vi "自动升级程序.vi"(8 "错误输入（无错误）":errorcluster) -> (0 "错误输出":errorcluster, 3 "确定":bool)   [LabVIEW 2016, in "数据传输系统-04.lvlib" / "自动更新.lvlib"]
uses:
  <vilib>/Utility/miscctls.llb/LVPointTypeDef.ctl
panel:
  out "自动下载倒计时/s":i32
  in  "滚动条":i32(c297)
  out "标题":string
  in  "取消":bool
  in  "确定":bool
  out "版本说明显示":string
  # "是否立即下载新版本(download right now)?"
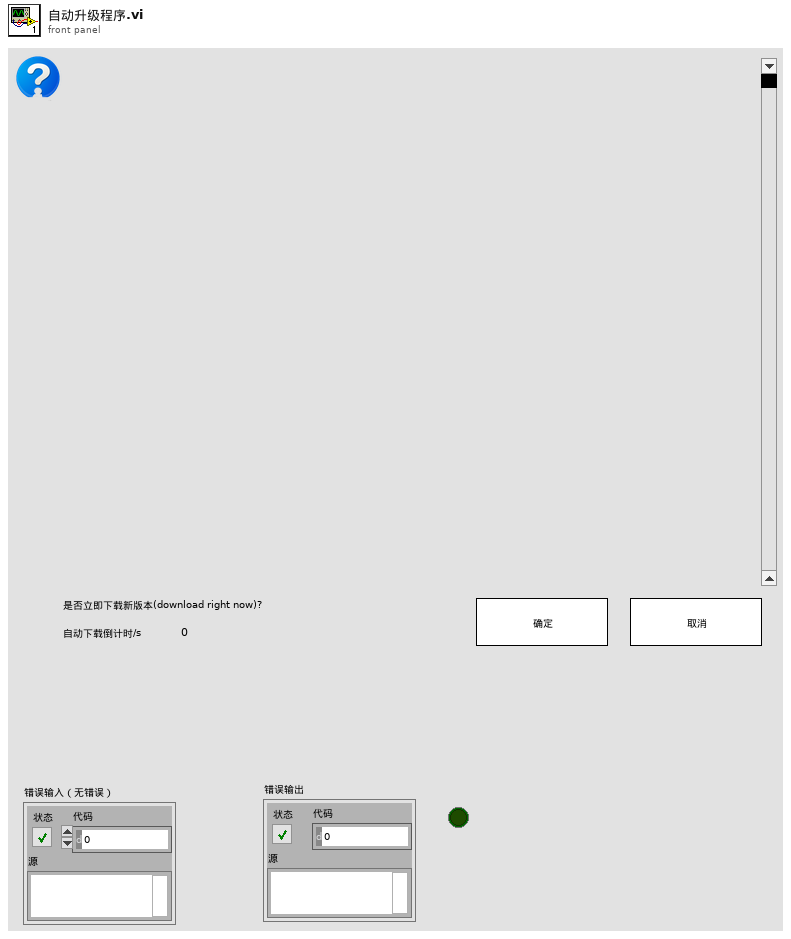
[diagram p1: front panel]
types:
  T1 = typedef "LVPointTypeDef.ctl" = cluster{"Horizontal":i16, "Vertical":i16}
  T2 = enum16{"open", "replace", "create", "open or create", "replace or create", "replace or create with confirmation"}
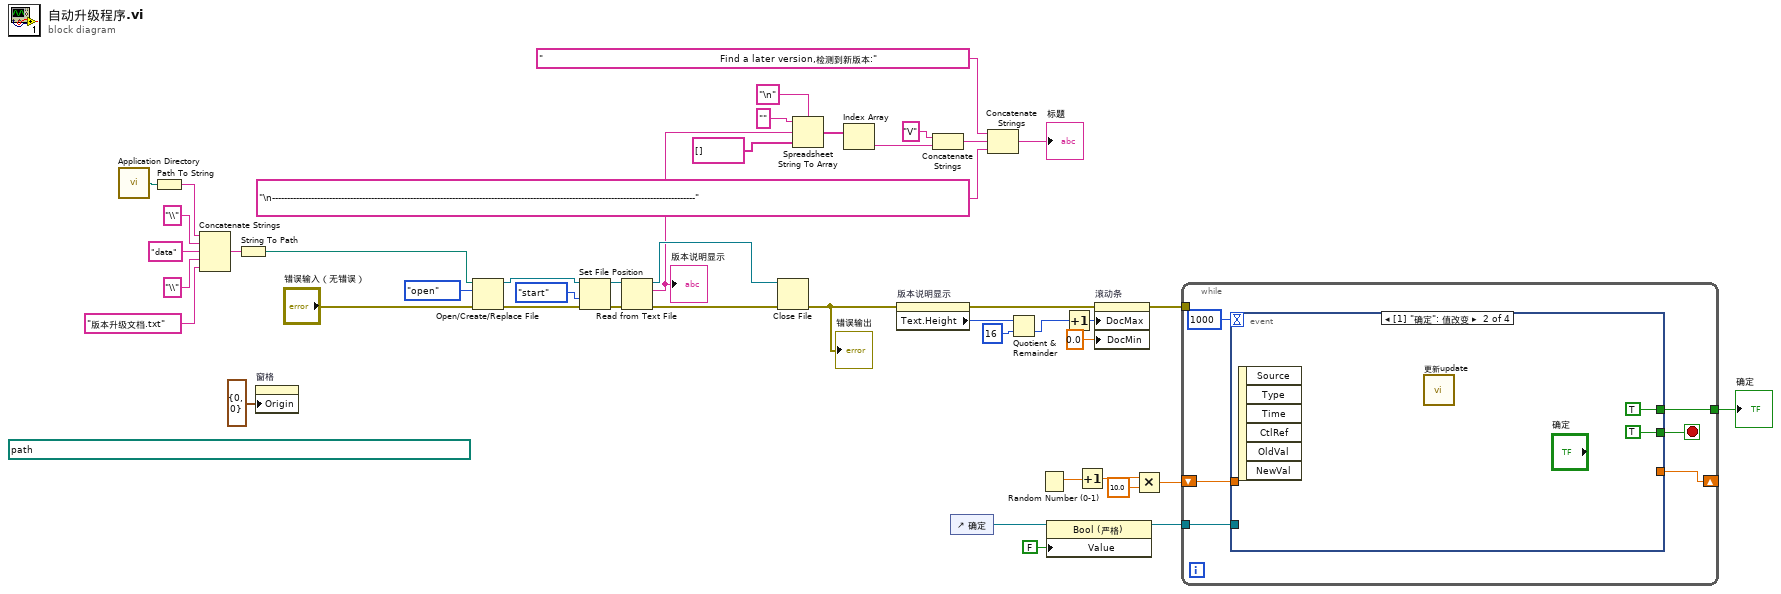
[diagram p0: block diagram]
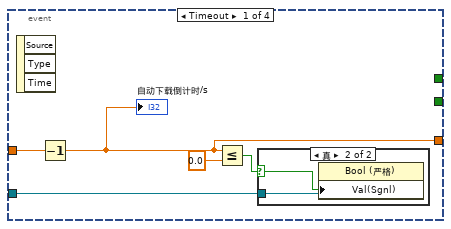
[diagram p2: hidden frame]
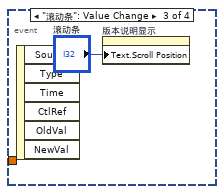
[diagram p4: hidden frame]
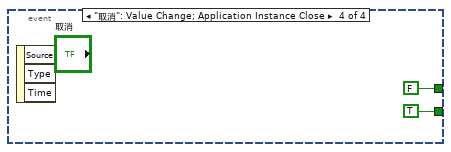
[diagram p5: hidden frame]
diagram:
  (unwired) path "F:/gitkraken/CC/平台数采程序 - V2.0.1（正式修改迭代版）/data/版本升级文档.txt" ("路径")
  n1 = call <vilib>:"Application Directory.vi"() -> ("Application Directory"=w33:path)
  n2 = Path To String(path=w33) -> (string=w36:string)
  n3 = Concatenate Strings(w36, "\\" ("字符串"), "data" ("字符串"), "\\" ("字符串"), "版本升级文档.txt" ("字符串")) -> (w30:string)
  n4 = String To Path(string=w30) -> (path=w9:path)
  n5 = property on="窗格" class="Pane"("Origin"=T1 {"Horizontal"=0, "Vertical"=0} ("原点")) -> ()  [unwired: 2 in, 2 out]
  n6 = Open/Create/Replace File(file path (use dialog)=w9, error in="错误输入（无错误）", operation (0:open)=T2."open" ("操作(0:open)")) -> (refnum out=w41:refnum<file>, error out=w40:errorcluster)  [unwired: 3 in, 1 out]
  n7 = Set File Position(refnum=w41, from (0:start)=enum16{"start", "end", "current"}."start" ("自（0:起始）"), error in=w40) -> (refnum out=w37:refnum<file>, error out=w39:errorcluster)  [unwired: 1 in]
  n8 = Read from Text File(file (use dialog)=w37, error in=w39) -> (refnum out=w43:refnum<file>, text=w25:string, error out=w44:errorcluster)  [unwired: 2 in, 1 out]
  "版本说明显示" <- w25
  n9 = Close File(refnum=w43, error in=w44) -> (error out=w11:errorcluster)  [unwired: 1 out]
  "错误输出" <- w11
  n10 = Spreadsheet String To Array(delimiter (Tab)="\n" ("分隔符(Tab)"), format string="" ("格式字符串"), spreadsheet string=w25, array type (2D Dbl)=string[] []) -> (array=w21:string[])
  n11 = Index Array(array=w21) -> (element=w20:string)  [unwired: 1 in]
  n12 = property on="版本说明显示" class="Str"(error in=w11) -> (error out=w12:errorcluster, "Text.Height"=w17:u32)  [unwired: 1 in, 1 out]
  n13 = Concatenate Strings("V" ("字符串"), w20) -> (w18:string)
  n14 = control-ref of="确定"() -> (w7:refnum<vi>)
  n15 = Concatenate Strings("                                                           Find a later version,检测到新版本:" ("标题"), w18, "\n---------------------------------------------------------------------------------------------------------------------------------------------" ("标题")) -> (→"标题":string)
  n16 = Quotient & Remainder(x=w17, y=u32 16) -> (floor(x/y)=w15:u32)  [unwired: 1 out]
  n17 = Random Number (0-1)() -> (number: 0 to 1=w2:dbl)
  n18 = property class="Bool (严格)"(reference=w7, "Value"=FALSE ("值")) -> (reference out=w6:refnum<vi>)  [unwired: 1 in, 1 out]
  n19 = Increment(x=w15) -> (x+1=w10:u32)
  n20 = Increment(x=w2) -> (x+1=w4:dbl)
  n21 = property on="滚动条" class="Scroll (严格)"(error in=w12, "DocMax"=w10, "DocMin"=0.0 ("滚动范围最小值")) -> (error out=w13:errorcluster)  [unwired: 1 in, 1 out]
  n22 = Multiply(x=w4, y=10.0) -> (x*y=w1:dbl)
  n23 = while {
    tunnel: [w50] -> w29
    tunnel: w13 -> [_]
    shift-right: [w47] -> _
    shift-left: w1 -> [w48]
    tunnel: w6 -> [w46]
    stop <- w51 stop-if-true
    n24 = event shown="[1] \"确定\": 值改变" {
      selector: _ -> [_ _ _ _]
      dyn-events: _ -> [_ _ _ _]
      timeout: 1000 -> [_ _ _ _]
      tunnel: [_ TRUE _ TRUE] -> w51
      tunnel: [_ TRUE ("确定") _ FALSE ("确定")] -> w50
      tunnel: w48 -> [w56 _ _ _]
      tunnel: [w55 _ _ _] -> w47
      tunnel: w46 -> [w53 _ _ _]
      event Timeout {
        n25 = event-data() -> ()  [unwired: 1 in, 3 out]
        n26 = Decrement(x=w56) -> (x-1=w55:dbl)
        "自动下载倒计时/s" <- w55
        n27 = Less Or Equal?(x=w55, y=0.0) -> (x <= y?=w54:bool)
        n28 = case shown="真" w54 {
          selector: w54 -> [_ w57]
          tunnel: w53 -> [_ w58]
          frame False {
          }
          frame True {
            n29 = property class="Bool (严格)"(reference=w58, "Val(Sgnl)"=w57) -> ()  [unwired: 1 in, 2 out]
          }
        }
      }
      event "确定": Value Change {
        n30 = event-data() -> ()  [unwired: 1 in, 6 out]
        n31 = call "更新update.vi"() -> ()  [unwired: 12 in]
      }
      event "滚动条": Value Change {
        n32 = event-data() -> ()  [unwired: 1 in, 6 out]
        n33 = property on="版本说明显示" class="Str"("Text.Scroll Position"="滚动条") -> ()  [unwired: 2 in, 2 out]
      }
      event "取消": Value Change; Application Instance Close {
        n34 = event-data() -> ()  [unwired: 1 in, 3 out]
      }
    }
  }
  "确定" <- w29
